vi "Unflatten.vi"(8 "error in":errorcluster, 10 "Type and Defs":variant, 11 "JSON in":refnum<class "JSON.lvclass">) -> (0 "error out":errorcluster, 2 "Data":variant, 3 "JSON out":refnum<class "JSON.lvclass">)   [LabVIEW 2017, in "Report_lib.lvlib" / "JSON.lvclass"]
doc: "This method serves for unflatten\ndata from JSON string"
uses:
  JSON.lvclass
  JSON.lvclass/JSON.ctl
  <vilib>/addons/_JKI.lib/Serialization/JSON/JKI JSON Serialization.lvlib
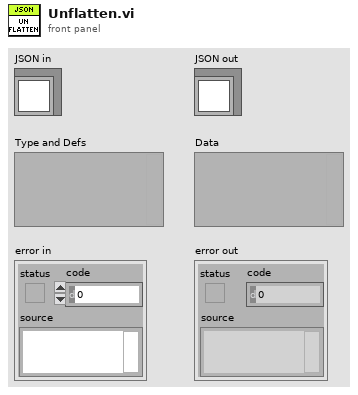
[diagram p1: front panel]
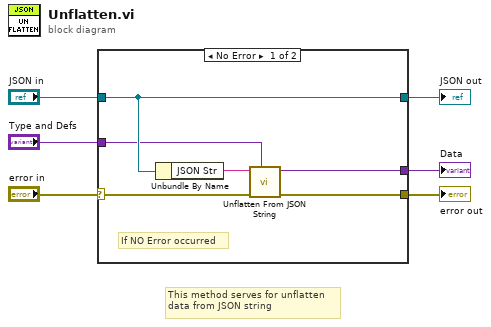
[diagram p0: block diagram]
diagram:
  # "This method serves for unflatten\ndata from JSON string"
  n1 = case shown="No Error" "error in" {
    selector: "error in" -> [w9 w14]
    tunnel: [w7 w14] -> w5
    tunnel: [w12 w13] -> w3
    tunnel: "JSON in" -> [w12 w13]
    tunnel: "Type and Defs" -> [w10 _]
    tunnel: [w8 _] -> w1
    frame No Error {
      # "If NO Error occurred"
      n2 = Unbundle By Name(w12) -> ("JSON Str"=w11:string)
      n3 = call <vilib>:"Unflatten From JSON String.vi"("Type and Defaults"=w10, "error in (no error)"=w9, "JSON String"=w11) -> ("error out"=w7:errorcluster, "Variant"=w8:variant)  [unwired: 7 in]
    }
    frame Error {
    }
  }
  "error out" <- w5
  "JSON out" <- w3
  "Data" <- w1
